vi "4_4.vi"() -> ()   [LabVIEW 2020]
panel:
  out "Output":i32[][](array[numeric])
  in  "Numeric":i32
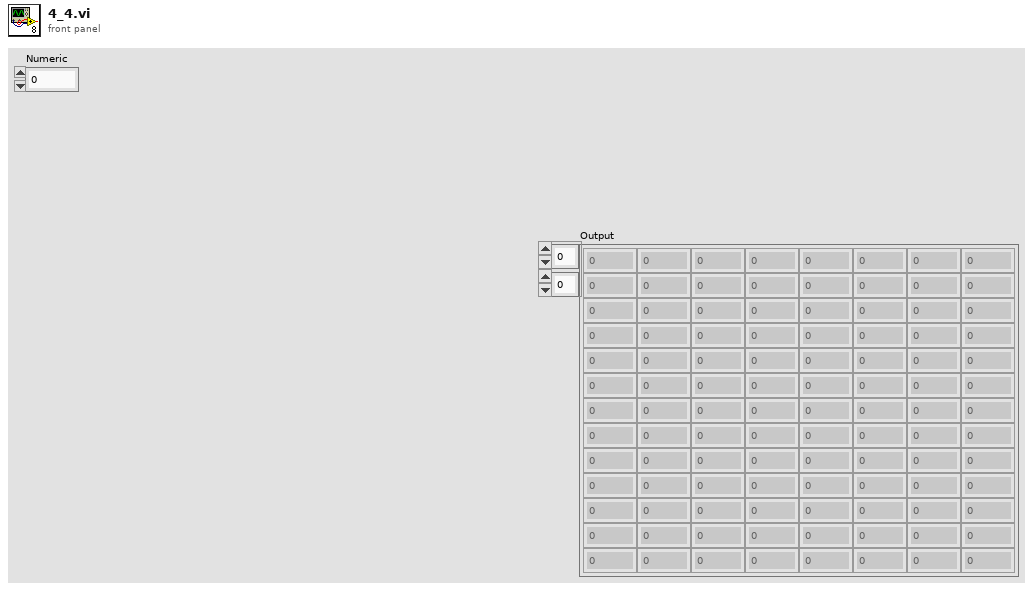
[diagram p1: front panel]
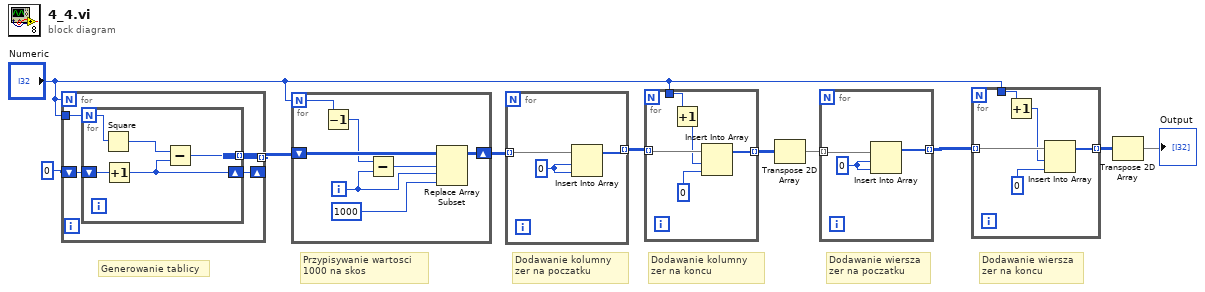
[diagram p0: block diagram]
diagram:
  # "Dodawanie wiersza\nzer na koncu"
  # "Dodawanie wiersza\nzer na poczatku"
  # "Dodawanie kolumny \nzer na koncu"
  # "Dodawanie kolumny \nzer na poczatku"
  # "Przypisywanie wartosci \n1000 na skos"
  # "Generowanie tablicy"
  n1 = for {
    N: "Numeric" -> [_]
    tunnel: "Numeric" -> [w14]
    tunnel: [w13] -> w9 mode=indexing
    shift-right: [w11] -> _
    shift-left: 0 -> [w12]
    n2 = for {
      N: w14 -> [w19]
      tunnel: [w17] -> w13 mode=indexing
      shift-right: [w15] -> w11
      shift-left: w12 -> [w16]
      n3 = Square(x=w19) -> (x^2=w18:i32)
      n4 = Increment(x=w16) -> (x+1=w15:i32)
      n5 = Subtract(x=w18, y=w15) -> (x-y=w17:i32)
    }
  }
  n6 = for {
    N: "Numeric" -> [w22]
    shift-right: [w26] -> w8
    shift-left: w9 -> [w25]
    i -> [w20]
    n7 = Decrement(x=w22) -> (x-1=w21:i32)
    n8 = Subtract(x=w21, y=w20) -> (x-y=w24:i32)
    n9 = Replace Array Subset(array=w25, new element=1000 ("new element/subarray"), index (row)=w24, index (col)=w20) -> (w26:i32[][])
  }
  n10 = for {
    tunnel: w8 -> [w29] mode=indexing
    tunnel: [w28] -> w7 mode=indexing
    w27 = 0 ("index")
    n11 = Insert Into Array(array=w29, index=w27, new element=w27) -> (w28:i32[])
  }
  n12 = for {
    tunnel: w7 -> [w34] mode=indexing
    tunnel: [w33] -> w6 mode=indexing
    tunnel: "Numeric" -> [w31]
    n13 = Increment(x=w31) -> (x+1=w30:i32)
    n14 = Insert Into Array(array=w34, index=w30, new element=0 ("index")) -> (w33:i32[])
  }
  n15 = Transpose 2D Array(2D array=w6) -> (transposed array=w4:i32[][])
  n16 = for {
    tunnel: w4 -> [w37] mode=indexing
    tunnel: [w36] -> w5 mode=indexing
    w35 = 0 ("index")
    n17 = Insert Into Array(array=w37, index=w35, new element=w35) -> (w36:i32[])
  }
  n18 = for {
    tunnel: w5 -> [w42] mode=indexing
    tunnel: [w41] -> w2 mode=indexing
    tunnel: "Numeric" -> [w39]
    n19 = Increment(x=w39) -> (x+1=w38:i32)
    n20 = Insert Into Array(array=w42, index=w38, new element=0 ("index")) -> (w41:i32[])
  }
  n21 = Transpose 2D Array(2D array=w2) -> (transposed array=→"Output":i32[][])
